vi "Vision Processing.vi"(4 "error in (no error)":errorcluster, 7 "Image Size":T1=enum."320x240") -> ()   [LabVIEW 2017]
doc: "This VI runs in parallel to other tasks. It gets images from the camera, processes them for color or shape and use that information to affect robot behavior."
uses:
  <vilib>/Rock Robotics/WPI/Camera/WPI_CameraImageSize.ctl
  Robot Global Data.vi
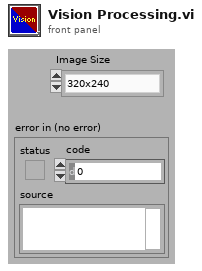
[diagram p1: front panel]
types:
  T1 = typedef "WPI_CameraImageSize.ctl" = enum16{"640x480", "320x240", "160x120", "Custom"}
  T2 = typedef "Image Type" = u32
  T3 = typedef "WPI_CameraDevRef.ctl" = cluster{"Camera Address":string, "CameraStatus":errorcluster}
  T4 = typedef "IMAQ Image.ctl" = refnum<image>
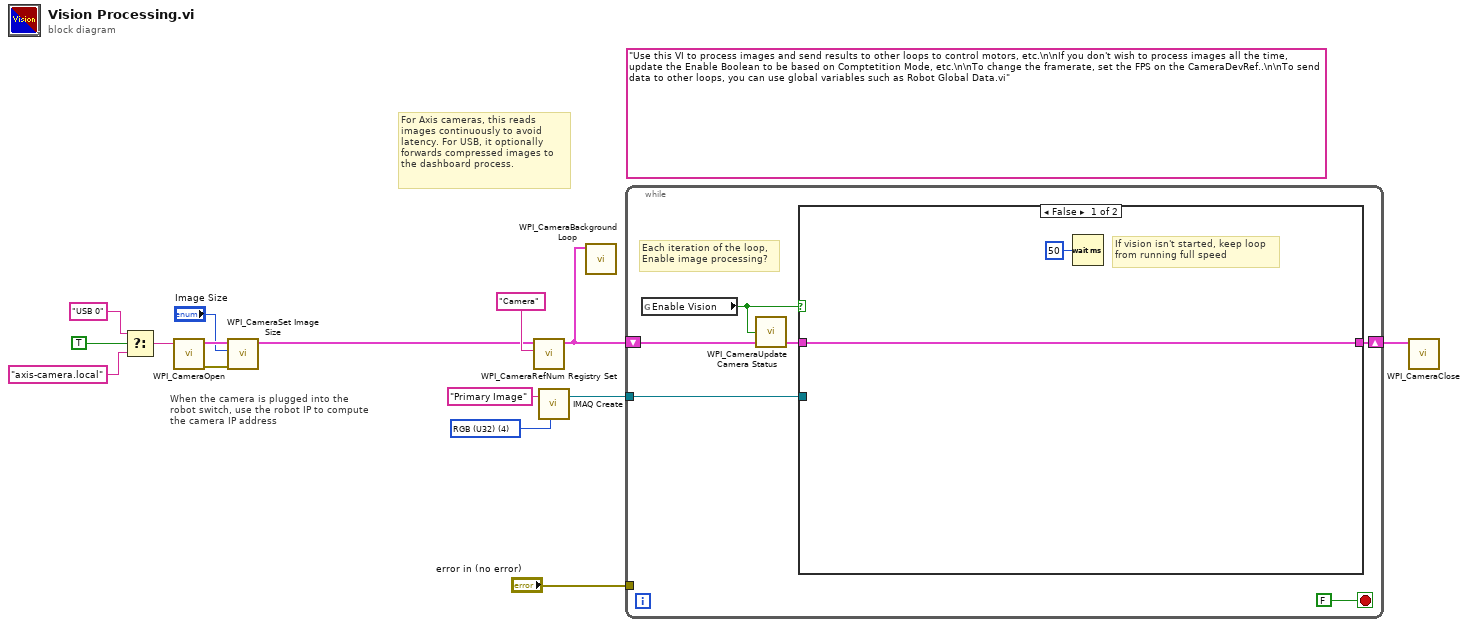
[diagram p0: block diagram]
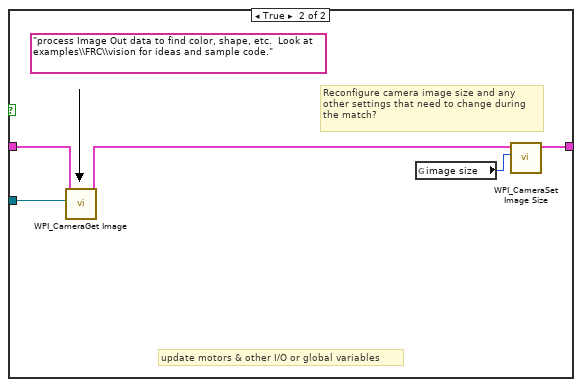
[diagram p2: hidden frame]
diagram:
  (unwired) "Use this VI to process images and send results to other loops to control motors, etc.\n\nIf you don't wish to process images all the time, update the Enable Boolean to be based on Comptetition Mode, etc.\n\nTo change the framerate, set the FPS on the CameraDevRef..\n\nTo send data to other loops, you can use global variables such as Robot Global Data.vi"
  w15 = T2 4 items=["Grayscale (U8)", "Grayscale (I16)", "Grayscale (SGL)", "Complex (CSG)", "RGB (U32)", "HSL (U32)", "RGB (U64)"] ("Image Type")
  # "When the camera is plugged into the\nrobot switch, use the robot IP to compute\nthe camera IP address"
  # "For Axis cameras, this reads\nimages continuously to avoid\nlatency. For USB, it optionally\nforwards compressed images to\nthe dashboard process."
  n1 = Select(t="USB 0" ("format string"), s=TRUE ("dot notation? (F)"), f="axis-camera.local" ("format string")) -> (s? t:f=w3:string)
  n2 = call <vilib>:"WPI_CameraOpen.vi"("Camera Address"=w3) -> ("error out"=w10:errorcluster, "CameraDevRef"=w11:T3)  [unwired: 1 in, 8 out]
  n3 = call <vilib>:"WPI_CameraSet Image Size.vi"("error in (no error)"=w10, "Image Size"="Image Size", "CameraDevRef"=w11) -> ("CameraDevRef Out"=w1:T3)  [unwired: 1 in, 7 out]
  n4 = call <vilib>:"WPI_CameraRefNum Registry Set.vi"("refnum name"="Camera", "CameraDevRef"=w1) -> ("CameraDevRef"=w9:T3)  [unwired: 2 in, 7 out]
  n5 = call "IMAQ Create"("Image Name"="Primary Image", "Image Type"=w15) -> ("New Image"=w13:T4)  [unwired: 2 in, 2 out]
  n6 = call <vilib>:"WPI_CameraBackground Loop.vi"("CameraDevRef"=w9) -> ()  [unwired: 11 in]
  n7 = while {
    shift-right: [w20] -> w7
    shift-left: w9 -> [w18]
    tunnel: w13 -> [w19]
    tunnel: "error in (no error)" -> [_]
    stop <- FALSE stop-if-true
    # "Each iteration of the loop,\nEnable image processing?"
    n8 = global read "Robot Global Data.vi" "Enable Vision"() -> (w16:bool)
    n9 = call <vilib>:"WPI_CameraUpdate Camera Status.vi"("CameraDevRef In"=w18, "Enable Vision"=w16) -> ("CameraDevRef Out"=w17:T3)  [unwired: 3 in]
    n10 = case shown="False" w16 {
      tunnel: w19 -> [_ w27]
      tunnel: [w23 w28] -> w20
      tunnel: w17 -> [w23 w25]
      frame False {
        # "If vision isn't started, keep loop\nfrom running full speed"
        n11 = Wait (ms)(milliseconds to wait=u32 50) -> ()  [unwired: 1 out]
      }
      frame True {
        (unwired) "process Image Out data to find color, shape, etc.  Look at examples\\FRC\\vision for ideas and sample code."
        # "update motors & other I/O or global variables"
        # "Reconfigure camera image size and any\nother settings that need to change during\nthe match?"
        n12 = call <vilib>:"WPI_CameraGet Image.vi"("Image"=w27, "CameraDevRef"=w25) -> ("CameraDevRef Out"=w24:T3)  [unwired: 1 in, 8 out]
        n13 = global read "Robot Global Data.vi" "image size"() -> (w26:T1)
        n14 = call <vilib>:"WPI_CameraSet Image Size.vi"("Image Size"=w26, "CameraDevRef"=w24) -> ("CameraDevRef Out"=w28:T3)  [unwired: 2 in, 7 out]
      }
    }
  }
  n15 = call <vilib>:"WPI_CameraClose.vi"("CameraDevRef"=w7) -> ()  [unwired: 1 in, 10 out]
